vi "Module Type.vi"(11 "DAQmxDI in":refnum<class "DAQmxDI.lvclass">) -> (2 "Module Type":string)   [LabVIEW 2020, in "VolatusDAQ.lvlib" / "DAQmxDI.lvclass"]
uses:
  DAQmxDI.lvclass
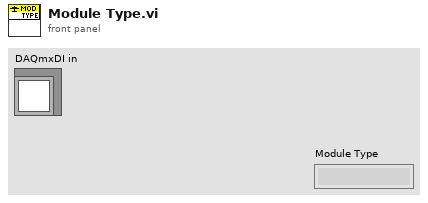
[diagram p1: front panel]
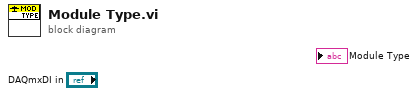
[diagram p0: block diagram]
diagram:
